vi "AOT.vi"(1 "height":dbl, 2 "base":dbl) -> (0 "output":dbl)   [LabVIEW 2017]
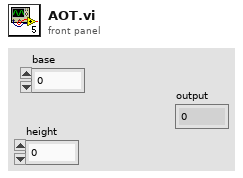
[diagram p1: front panel]
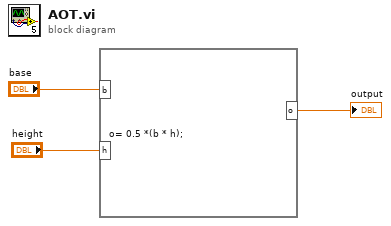
[diagram p0: block diagram]
diagram:
  n1 = formula code="o= 0.5 *(b * h);"("h"="height", "b"="base") -> ("o"=→"output":dbl)
